vi "tipshaping.vi"(8 "error in (no error)":errorcluster, 11 "Input":string="34,45,89") -> (0 "error out":errorcluster, 3 "Output":string)   [LabVIEW 2014]
uses:
  <userlib>/Nanonis Prog Interface V5/Nanonis Prog Interface.lvlib
panel:
  in  "milliseconds to wait":u32
  out "size(s)":i32=3
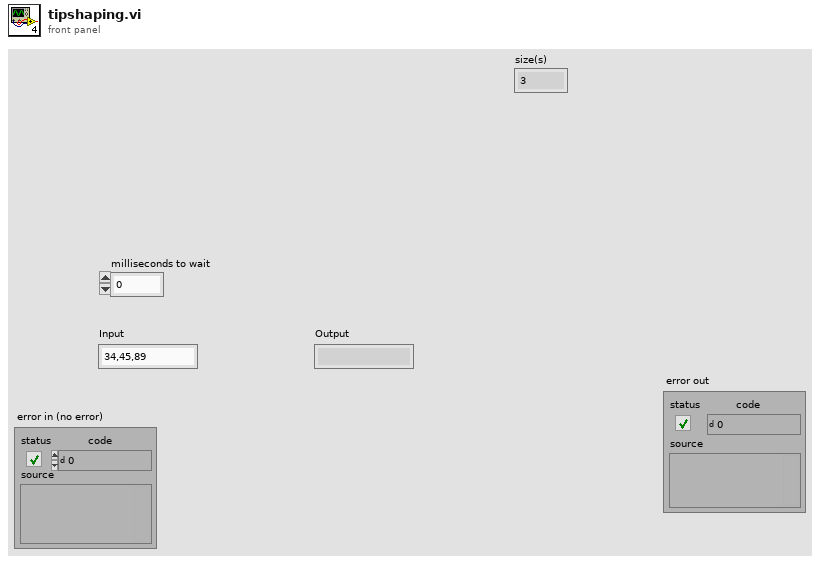
[diagram p1: front panel]
types:
  T1 = cluster{"TipLift":dbl, "Bias Settling Time":dbl, "Lift Height":dbl, "Lift Time 2":dbl, "Lifting Bias":dbl, "Lift Time 1":dbl}
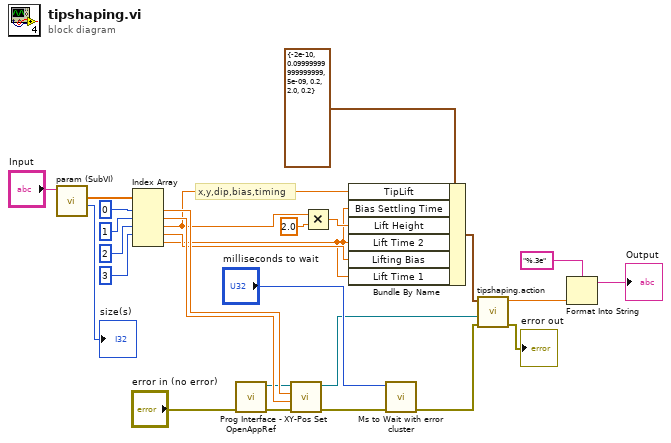
[diagram p0: block diagram]
diagram:
  # "x,y,dip,bias,timing"
  n1 = call <userlib>:"param (SubVI).vi"("Input"="Input") -> ("num"=→"size(s)":i32, "parm"=w25:dbl[])  [unwired: 8 in, 1 out]
  n2 = Index Array(array=w25, index #1=0 ("index"), index #2=1 ("index"), index #3=2 ("index"), index #4=3 ("index")) -> (element #1=w14:dbl, element #2=w13:dbl, element #3=w9:dbl, element #4=w6:dbl, element #5=w5:dbl)  [unwired: 1 in]
  n3 = call <userlib>:"Prog Interface - OpenAppRef.vi"("Error in (no error)"="error in (no error)") -> ("Error out"=w11:errorcluster, "Application reference"=w12:refnum<vi>)  [unwired: 5 in]
  n4 = call <userlib>:"XY-Pos Set.vi"("error in (no error)"=w11, "Y (m)"=w13, "X (m)"=w14, "Application ref in"=w12) -> ("error out"=w3:errorcluster, "Application ref out"=w1:refnum<vi>)  [unwired: 4 in]
  n5 = Multiply(x=w9, y=2.0) -> (x*y=w8:dbl)
  n6 = Bundle By Name(cluster=T1 {"TipLift"=-2e-10, "Bias Settling Time"=0.09999999999999999, "Lift Height"=5e-09, "Lift Time 2"=0.2, "Lifting Bias"=2.0, "Lift Time 1"=0.2} ("TipShapingParam"), "TipLift"=w9, "Bias Settling Time"=w5, "Lift Height"=w8, "Lift Time 2"=w5, "Lifting Bias"=w6, "Lift Time 1"=w5) -> (w15:T1)
  n7 = call <userlib>:"Ms to Wait with error cluster.vi"("error in (no error)"=w3, "milliseconds to wait"="milliseconds to wait") -> ("error out"=w4:errorcluster)  [unwired: 4 in, 1 out]
  n8 = call <userlib>:"tipshaping.action.vi"("Error in (no error)"=w4, "Application reference"=w1, "TipShapingParam"=w15) -> ("error out"=→"error out":errorcluster, "dz"=w18:sgl)  [unwired: 7 in]
  n9 = Format Into String(format string="%.3e", w18) -> (resulting string=→"Output":string)  [unwired: 2 in, 1 out]
